vi "Class - Get Accessors.vi"(7 "Msg Chain":string, 8 "error in (no error)":errorcluster {"code" format="Error %.0f"}, 10 "Classes":refnum<class "Class Documentation.lvclass">[](array[class]), 11 "VIDoc Printer - Confluence In":refnum<class "VIDoc Printer - Confluence.lvclass">) -> (0 "error out":errorcluster {"code" format="Error %.0f"}, 3 "VIDoc Printer - Confluence Out":refnum<class "VIDoc Printer - Confluence.lvclass">)   [LabVIEW 2023, in "VIDoc Printer - Confluence.lvlib" / "VIDoc Printer - Confluence.lvclass"]
uses:
  VIDoc Printer - Confluence.lvclass
  C:/projects/DMC/GitHub/DMC CLI VIDoc/Source/Documentation Generation/Printers/Printer/VIDoc Printer.lvclass
  Parsing/Class Documentation/Class Documentation.lvclass
  Parsing/Class Documentation/Class Documentation.lvclass/Class Documentation.ctl
  Printer/VIDoc Printer.lvclass/VIDoc Printer.ctl
  Parsing/TypeDefs/VI Type Extended Enum.ctl
  Confluence Formatting/Types/Format Combo Box.ctl
  Types/VI Method Types.ctl
  VIDoc Printer - Confluence.lvclass/VIDoc Printer - Confluence.ctl
  Accessors/Get Class Get Accessors Expand.vi
  Printer/Accessors/Get Class Settings - Get Accessors Scope.vi
  Printer/Accessors/Get Class Settings - Get Accessor Detail Level.vi
  Parsing/Class Documentation/Get Methods.vi
  Parsing/Class Documentation/Get Name.vi
  Printer/VIDoc Printer.lvclass
  UI Interaction/UI Interaction.lvclass
  Parsing/VIDoc Parsing.lvlib
  Confluence Formatting/Confluence Formatting.lvlib
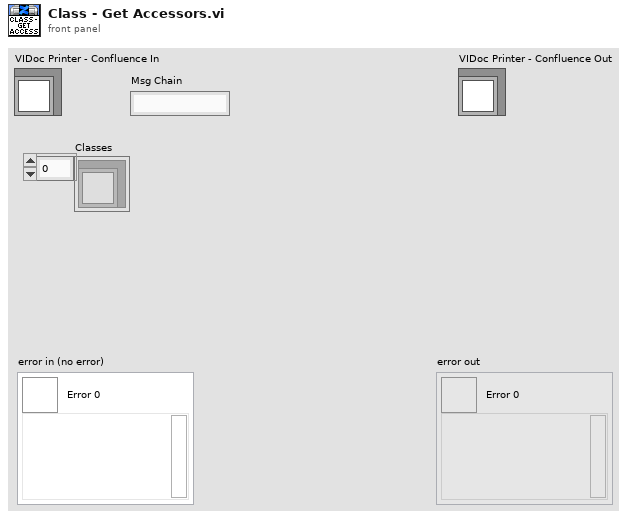
[diagram p1: front panel]
types:
  T1 = typedef "VIDoc Parsing.lvlib/VI Type Extended Enum.ctl" = enum16{"Unknown", "Class Method", "Class Accessor Get", "Class Accessor Set", "Class Control", "Library Method", "Library Control", "VI", "Control"}
  T2 = typedef "VIDoc Printer - Confluence.lvlib/VIDoc Printer - Confluence.lvclass/VI Method Types.ctl" = enum16{"Library", "Class", "Interface", "LLB", "UI", "List"}
  T3 = typedef "Confluence Formatting.lvlib/Format Combo Box.ctl" = string
  T4 = typedef "VIDoc Parsing.lvlib/Method Spec Cluster.ctl" = cluster{"VI Type Ext":T1, "Name":string, "Path":path, "Get Conpane Image":T5, "Description":string, "Get Library Access Scope":enum32{"invalid scope", "public", "private", "protected", "community"}, "Dispatch":T6, "ContainsCompiledCode":bool, "Exec.IsReentrant":bool, "Exec.ReentrancyType":enum16{"Share clones between instances", "Preallocate clone for each instance"}, "ExecInlining":bool, "ExecInlineIfPossible":bool, "Auto Err Handling":bool, "CodeComplexity":sgl, "Bookmark Tags":string[], "Control VI Type":enum32{"not a control VI", "control", "typedef", "strict typedef"}, "Controls":T7[], "VI Type":enum32{"invalid VI type", "Standard VI", "Control VI", "Global VI", "Polymorphic VI", "Configuration VI", "SubSystem", "Facade VI", "Method VI", "Statechart Diagram VI"}, "Minimum Size":T9, "Front Panel Window:Title":string, "Front Panel Window:Behavior":enum32{"Invalid", "Default", "Floating", "Floating/Auto-Hide", "Modal"}, "Front Panel Window:Closeable":bool, "Must Override":bool, "Must Use Parent Implementation":bool, "VI Icon":T5, "Front Panel":T5, "History:Revision Number":u32, "Metrics:Total Data Size":u32, "Execution:Allow Debugging":bool, "Execution:Preferred Exec System":enum32{"invalid execution system", "user interface", "standard", "instrument i/o", "data acquisition", "other 1", "other 2", "same as caller"}, "Execution:Priority":enum32{"invalid priority", "background priority", "normal priority", "above normal priority", "high priority", "time critical priority", "subroutine"}, "BM Tag Text":string[], "Block Diagram":T5, "Structure Tree":T10[]}
  T5 = typedef "imagedata.ctl" = cluster{"image type":i32, "image depth":i32, "image":u8[], "mask":u8[], "colors":u32[], "Rectangle":cluster{"left":i16, "top":i16, "right":i16, "bottom":i16}}
  T6 = typedef "VIDoc Parsing.lvlib/Class Dispatch Type Enum.ctl" = enum16{"None", "Static", "Dynamic"}
  T7 = typedef "VIDoc Parsing.lvlib/Controls Info Cluster.ctl" = cluster{"Name":string, "Description":string, "Data Type":string, "Tip Strip":string, "UID":i32, "Image Data":T5, "ToggleKeyBind":T8, "Raw Label":string, "Raw Caption":string}
  T8 = typedef "LVKeyTypeDef.ctl" = cluster{"Focus":bool, "Control":bool, "Shift":bool, "Key":string}
  T9 = typedef "LVPointTypeDef.ctl" = cluster{"Horizontal":i16, "Vertical":i16}
  T10 = typedef "VIDoc Parsing.lvlib/Structure Reporter.lvlib/Tree Cluster.ctl" = cluster{"Object Class Name":string, "Labels":string[], "Child Tag":string, "Item Indent":i32, "Child Only?":bool, "Glyph Index":i32}
  T11 = typedef "VIDoc Printer.lvlib/Printer Settings.lvclass/Scope Settings.ctl" = cluster{"Public":bool, "Protected":bool, "Community":bool, "Private":bool, "Unknown":bool}
  T12 = typedef "VIDoc Printer.lvlib/Printer Settings.lvclass/Detail Level Enum.ctl" = enum16{"None", "Minimal", "Standard", "Full"}
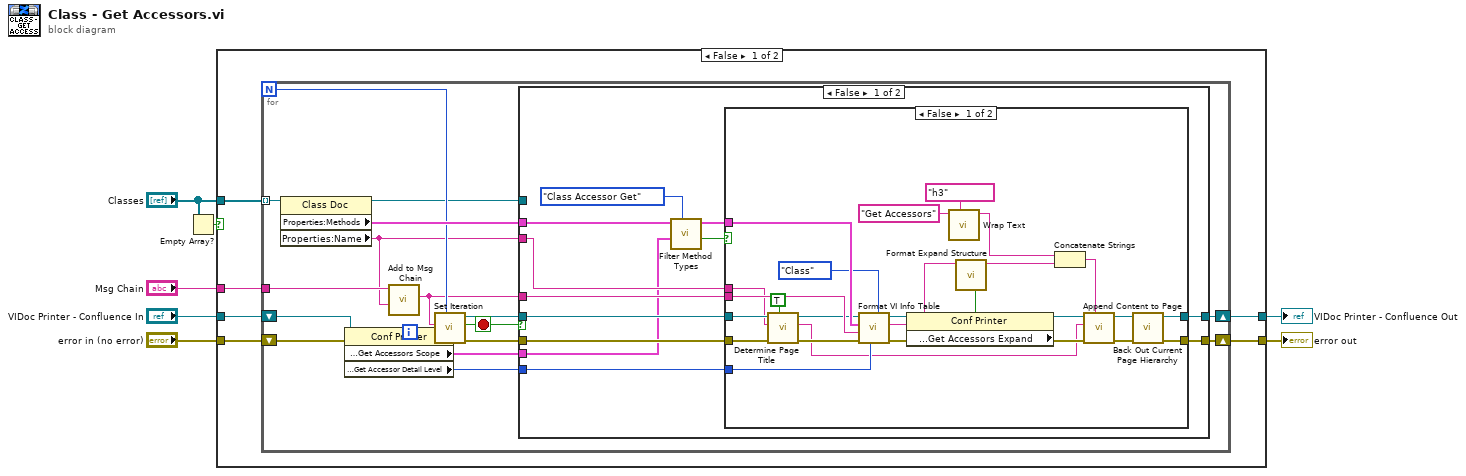
[diagram p0: block diagram]
diagram:
  n1 = Empty Array?(array="Classes") -> (empty?=w7:bool)
  n2 = case shown="False" w7 {
    tunnel: [w13 w74] -> w6
    tunnel: [w12 w75] -> w5
    tunnel: "error in (no error)" -> [w11 w74]
    tunnel: "Classes" -> [w10 _]
    tunnel: "VIDoc Printer - Confluence In" -> [w9 w75]
    tunnel: "Msg Chain" -> [w8 _]
    frame False {
      n3 = for {
        N -> [w25]
        shift-right: [w30] -> w13
        shift-left: w11 -> [w28]
        shift-right: [w31] -> w12
        shift-left: w9 -> [w18]
        tunnel: w10 -> [w32] mode=indexing
        tunnel: w8 -> [w23]
        i -> [w24]
        stop <- w21 stop-if-true
        n4 = property class="Class Doc"(reference=w32) -> (reference out=w20:refnum<class "Class Documentation.lvclass">, "Properties:Methods"=w29:T4[], "Properties:Name"=w22:string)  [unwired: 1 in, 1 out]
        n5 = property class="Conf Printer"(reference=w18, error in=w28) -> (reference out=w17:refnum<class "VIDoc Printer - Confluence.lvclass">, error out=w19:errorcluster, "Properties:Settings:Classes:Get Accessors Scope"=w15:T11, "Properties:Settings:Classes:Get Accessor Detail Level"=w14:T12)
        n6 = call "Add to Msg Chain.vi"("New"=w22, "Msg Chain in"=w23) -> ("Msg Chain out"=w16:string)  [unwired: 9 in]
        n7 = call "Set Iteration.vi"("Progress Max"=w25, "error in (no error)"=w19, "Progress Value"=w24, "Message (No Message Update)"=w16, "VIDoc Printer In"=w17) -> ("error out"=w26:errorcluster, "Abort?"=w21:bool, "VIDoc Printer Out"=w27:refnum<class "VIDoc Printer - Confluence.lvclass">)  [unwired: 4 in]
        n8 = case shown="False" w21 {
          tunnel: [w44 w72] -> w31
          tunnel: [w43 w73] -> w30
          tunnel: w29 -> [w38 _]
          tunnel: w27 -> [w41 w72]
          tunnel: w26 -> [w42 w73]
          tunnel: w22 -> [w39 _]
          tunnel: w20 -> [_ _]
          tunnel: w16 -> [w40 _]
          tunnel: w15 -> [w34 _]
          tunnel: w14 -> [w33 _]
          frame False {
            n9 = call "Filter Method Types.vi"("VI Type to filter for"=VI_Type_Extended_Enum."Class Accessor Get" ("y"), "Scope"=w34, "Methods"=w38) -> ("All Filtered?"=w36:bool, "Filtered Methods"=w37:T4[])  [unwired: 6 in, 1 out]
            n10 = case shown="False" w36 {
              tunnel: [w51 w71] -> w44
              tunnel: [w49 w70] -> w43
              tunnel: w42 -> [w58 w70]
              tunnel: w41 -> [w59 w71]
              tunnel: w40 -> [w63 _]
              tunnel: w33 -> [w62 _]
              tunnel: w37 -> [w60 _]
              tunnel: w39 -> [w54 _]
              frame False {
                n11 = call "Determine Page Title.vi"("Update Current Page (F)"=TRUE, "error in (no error)"=w58, "Name"=w54, "VIDoc Printer - Confluence In"=w59) -> ("error out"=w57:errorcluster, "Page Title"=w53:string, "VIDoc Printer - Confluence Out"=w56:refnum<class "VIDoc Printer - Confluence.lvclass">)  [unwired: 4 in, 1 out]
                n12 = call "Format VI Info Table.vi"("Type"=VI_Method_Types."Class", "Methods"=w62, "Error in"=w57, "Msg Chain"=w63, "VI Info Array"=w60, "VIDoc Printer - Confluence In"=w56) -> ("Error out"=w65:errorcluster, "Table String"=w61:string, "VIDoc Printer - Confluence Out"=w64:refnum<class "VIDoc Printer - Confluence.lvclass">)  [unwired: 3 in]
                n13 = property class="Conf Printer"(reference=w64) -> (reference out=w47:refnum<class "VIDoc Printer - Confluence.lvclass">, "Properties:Expand?:Class:Get Accessors Expand"=w46:bool)  [unwired: 1 in, 1 out]
                n14 = call "Wrap Text.vi"("Formatting"=T3 "h3", "String"="Get Accessors") -> ("Wrapped String"=w67:string)  [unwired: 8 in, 1 out]
                n15 = call "Format Expand Structure.vi"("Enable? (T)"=w46, "Content"=w61) -> ("Expand String"=w48:string)  [unwired: 8 in, 1 out]
                n16 = Concatenate Strings(w67, w48) -> (w66:string)
                n17 = call "Append Content to Page.vi"("Page Content"=w66, "error in (no error)"=w65, "Page Title"=w53, "VIDoc Printer - Confluence In"=w47) -> ("error out"=w50:errorcluster, "VIDoc Printer - Confluence Out"=w52:refnum<class "VIDoc Printer - Confluence.lvclass">)  [unwired: 6 in]
                n18 = call "Back Out Current Page Hierarchy.vi"("error in (no error)"=w50, "VIDoc Printer - Confluence In"=w52) -> ("error out"=w49:errorcluster, "VIDoc Printer - Confluence Out"=w51:refnum<class "VIDoc Printer - Confluence.lvclass">)  [unwired: 8 in]
              }
              frame True {
              }
            }
          }
          frame True {
          }
        }
      }
    }
    frame True {
    }
  }
  "error out" <- w6
  "VIDoc Printer - Confluence Out" <- w5
